vi "FPGA_NI_meter.vi"() -> ()   [LabVIEW 2024]
uses:
  <vilib>/eio/EIONode/EIONode.xnode
  <vilib>/rvi/eio/common/nirviEmuTemplateMethod_errors.vi
  <vilib>/platform/TimedLoop/XDataNode/XDataNode.xnode
  <vilib>/Platform/TimedLoop/XDataNode/nitl_modes.ctl
  <vilib>/Platform/TimedLoop/XDataNode/XDNodeRunTimeDep.lvlib
  <vilib>/Platform/TimedLoop/XDataNode/wakeup.ctl
  <vilib>/Platform/TimedLoop/XDataNode/timing_clust.ctl
panel:
  out "ch2":fxp<+/-,32,7>[](array[numeric])
  out "ch1":fxp<+/-,32,7>[](array[numeric])
  out "ch0":fxp<+/-,32,7>[](array[numeric])
  in  "nSamples":i32=50
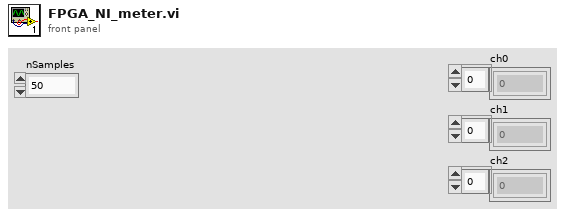
[diagram p1: front panel]
types:
  T1 = typedef "XDNodeRunTimeDep.lvlib/timing_clust.ctl" = cluster{"Expected End [f-1]":u64, "Actual End [f-1]":u64, "Finished Late? [f-1]":bool, "Expected End [i-1]":u64, "Actual End [i-1]":u64, "Finished Late? [i-1]":bool, "Expected Start [i]":u64, "Actual Start [i]":u64, "Expected Start [f]":u64, "Actual Start [f]":u64, "Source Name":string, "Structure Name":string, "Period":i64, "Deadline":i64, "Offset":i64, "Start":i64, "Priority":i32, "Timeout":i32, "Mode":T2, "Wakeup Reason":T3, "Error":errorcluster, "Source Type":string, "Secondary Source Type":string, "Global End Time":u64, "Global Start Time":u64, "Frame Duration":u64, "Iteration Duration":u64, "Assigned CPU":i32, "I/O Scan Engine Mode":u32}
  T2 = typedef "XDNodeRunTimeDep.lvlib/nitl_modes.ctl" = enum32{"No Change", "Process missed periods, maintain original phase", "Discard missed periods, maintain original phase", "Process missed periods, ignore original phase", "Discard missed periods, ignore original phase"}
  T3 = typedef "XDNodeRunTimeDep.lvlib/wakeup.ctl" = enum32{"Normal", "Aborted", "Asynchronous wakeup", "Timing source error", "Timed loop error", "Timeout"}
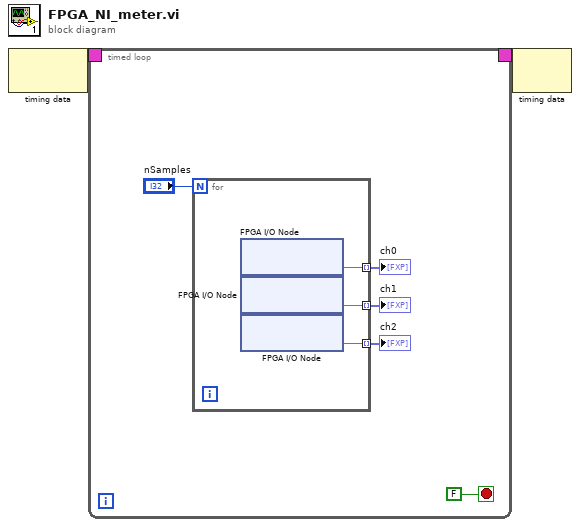
[diagram p0: block diagram]
diagram:
  n1 = node-c288() -> (w2:T1)  [unwired: 1 in]
  n2 = timed-loop {
    timing: w2 -> [_]
    timing-out: [_] -> w1
    stop <- FALSE stop-if-true
    n3 = for {
      N: "nSamples" -> [_]
      tunnel: [w10] -> w5 mode=indexing
      tunnel: [w9] -> w4 mode=indexing
      tunnel: [w8] -> w3 mode=indexing
      n4 = xnode "FPGA I/O Node"() -> ("Mod1/CH0"=w10:fxp<+/-,32,7>)  [unwired: 1 in, 1 out]
      n5 = xnode "FPGA I/O Node"() -> ("Mod1/CH1"=w9:fxp<+/-,32,7>)  [unwired: 1 in, 1 out]
      n6 = xnode "FPGA I/O Node"() -> ("Mod1/CH2"=w8:fxp<+/-,32,7>)  [unwired: 1 in, 1 out]
    }
    "ch0" <- w5
    "ch1" <- w4
    "ch2" <- w3
  }
  n7 = node-c288(w1) -> ()  [unwired: 1 out]
